vi "Get Todo Bookmarks.vi"(6 "open VI references? (False)":bool, 8 "error in (no error)":errorcluster, 11 "Directory to Search":path) -> (0 "error out":errorcluster, 2 "todo bookmarks":map{path, T1}(c390))   [LabVIEW 2020]
uses:
  <vilib>/Utility/miscctls.llb/LVBookmarkInfoTypeDef.ctl
  af485d53-b5a2-4225-9b29-f30f09fd7990.vi
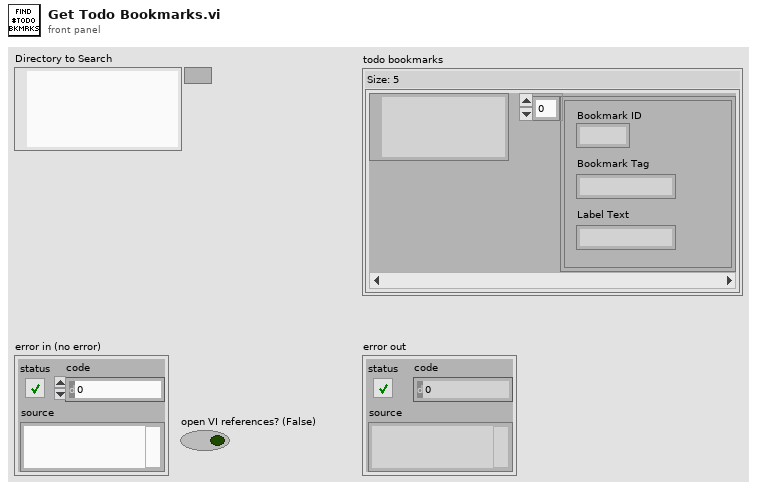
[diagram p1: front panel]
types:
  T1 = typedef "LVBookmarkInfoTypeDef.ctl" = cluster{"Bookmark ID":u32, "Bookmark Tag":string, "Label Text":string}[]
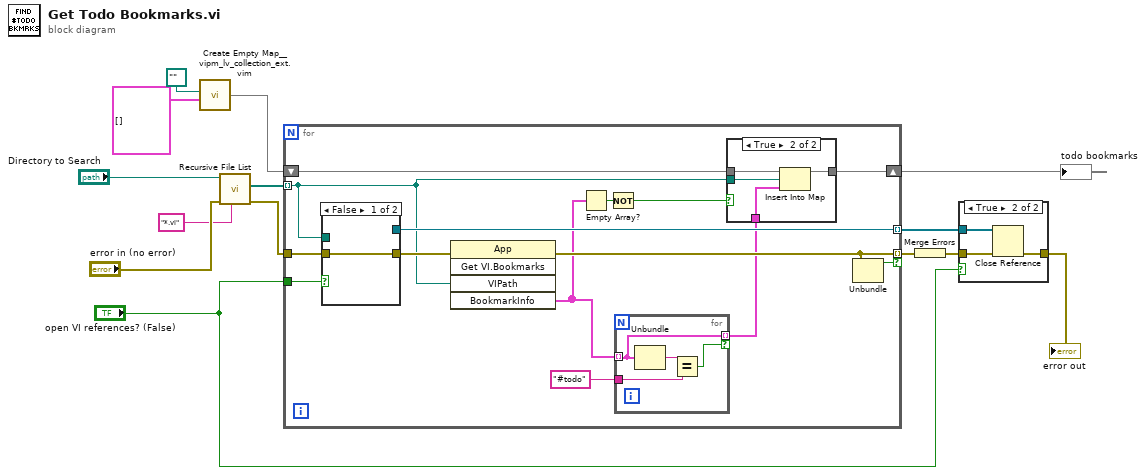
[diagram p0: block diagram]
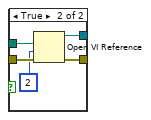
[diagram p3: hidden frame]
diagram:
  n1 = call "Create Empty Map__vipm_lv_collection_ext.vim"("value type"=T1 [] ("Bookmark Information"), "key type"=path "" ("VI Path")) -> ("empty map"=w9:map{path, T1})  [unwired: 8 in]
  n2 = call <vilib>:"Recursive File List.vi"("pattern"="*.vi", "error in (no error)"="error in (no error)", "Folder Path"="Directory to Search") -> ("error out"=w12:errorcluster, "All Files in Dir"=w4:path[])  [unwired: 4 in, 3 out]
  n3 = for {
    tunnel: w4 -> [w24] mode=indexing
    tunnel: [w27] -> w5 mode=indexing
    shift-right: [w25] -> w14
    shift-left: w9 -> [w18]
    tunnel: w12 -> [w26]
    tunnel: [w22] -> w6 mode=indexing if=w21
    tunnel: "open VI references? (False)" -> [w15]
    n4 = case shown="False" w15 {
      tunnel: [w29 w34] -> w28
      tunnel: [_ w33] -> w27
      tunnel: w26 -> [w29 w32]
      tunnel: w24 -> [_ w30]
      frame False {
      }
      frame True {
        n5 = Open VI Reference(vi path=w30, options=2, error in (no error)=w32) -> (vi reference=w33:refnum<vi>, error out=w34:errorcluster)  [unwired: 3 in]
      }
    }
    n6 = invoke class="App" method="Get VI.Bookmarks"(error in=w28, "VIPath"=w24) -> (error out=w22:errorcluster, "BookmarkInfo"=w17:T1)  [unwired: 3 in, 3 out]
    n7 = Empty Array?(array=w17) -> (empty?=w23:bool)
    n8 = Not(x=w23) -> (.not. x?=w20:bool)
    n9 = for {
      tunnel: w17 -> [w36] mode=indexing
      tunnel: "#todo" ("Bookmark Tag") -> [w37]
      tunnel: [w36] -> w16 mode=indexing if=w35
      n10 = Unbundle(w36) -> ("Bookmark Tag"=w38:string)  [unwired: 2 out]
      n11 = Equal?(x=w38, y=w37) -> (x = y?=w35:bool)
    }
    n12 = case shown="True" w20 {
      tunnel: w18 -> [w39 w43]
      tunnel: [w39 w42] -> w25
      tunnel: w24 -> [_ w41]
      tunnel: w16 -> [_ w40]
      frame False {
      }
      frame True {
        n13 = Insert Into Map(map in=w43, key=w41, value=w40) -> (map out=w42:map{path, T1})  [unwired: 2 out]
      }
    }
    n14 = Unbundle(w22) -> ("status"=w21:bool)  [unwired: 2 out]
  }
  "todo bookmarks" <- w14
  n15 = Merge Errors(w6) -> (w11:errorcluster)
  n16 = case shown="True" "open VI references? (False)" {
    tunnel: w11 -> [w44 w47]
    tunnel: [w44 w46] -> w10
    tunnel: w5 -> [_ w45]
    frame False {
    }
    frame True {
      n17 = Close Reference(reference=w45, error in (no error)=w47) -> (error out=w46:errorcluster)
    }
  }
  "error out" <- w10
